vi "Get WS Status.vi"(4 "Secret ID (Default)":string, 6 "Access ID (Default)":string, 7 "WS Name":string, 8 "error in (no error)":errorcluster, 9 "Port":u16, 10 "Host":string, 11 "Scheme (HTTP)":T2) -> (0 "error out":errorcluster, 3 "Status":T1)   [LabVIEW 2020, in "WS Admin.lvlib"]
uses:
  WS Admin.lvlib
  Scheme.ctl
  WS Status.ctl
  Client Data.ctl
  HTTP Method.ctl
  <vilib>/regexp/Match Regular Expression.xnode
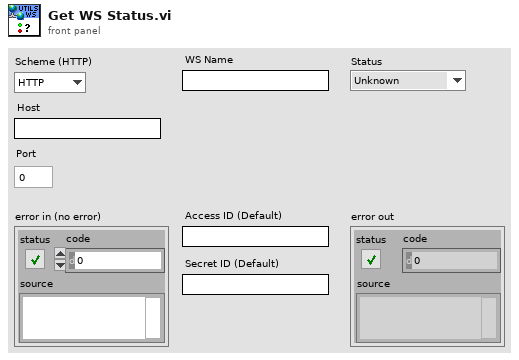
[diagram p1: front panel]
types:
  T1 = typedef "WS Admin.lvlib/WS Status.ctl" = enum16{"Unknown", "Paused", "Running"}
  T2 = typedef "WS Admin.lvlib/Scheme.ctl" = enum16{"HTTP", "HTTPS"}
  T3 = typedef "WS Admin.lvlib/HTTP Method.ctl" = enum16{"GET", "POST", "PUT", "DELETE"}
  T4 = typedef "WS Admin.lvlib/Client Data.ctl" = cluster{"HTTP Method":T3, "URL Path":string, "Access ID":string, "Secret ID":string}
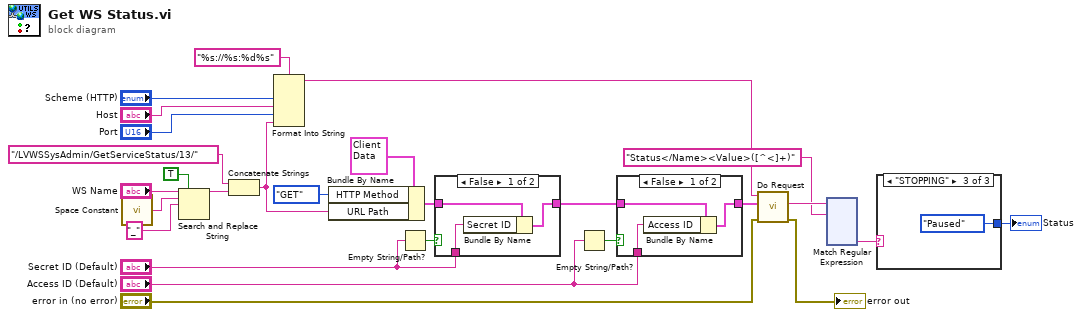
[diagram p0: block diagram]
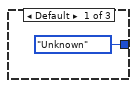
[diagram p2: hidden frame]
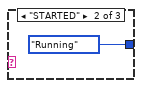
[diagram p3: hidden frame]
diagram:
  n1 = call <vilib>:"Space Constant.vi"() -> ("String"=w26:string)
  n2 = Search and Replace String(replace all?=TRUE ("replace all? (F)"), input string="WS Name", search string=w26, replace string="_" ("replace string (\"\")")) -> (result string=w19:string)  [unwired: 4 in, 3 out]
  n3 = Concatenate Strings("/LVWSSysAdmin/GetServiceStatus/13/", w19) -> (w16:string)
  n4 = Format Into String(format string="%s://%s:%d%s", "Scheme (HTTP)", "Host", "Port", w16) -> (resulting string=w6:string)  [unwired: 2 in, 1 out]
  n5 = Bundle By Name(cluster=T4 {"HTTP Method"=enum."GET", "URL Path"="", "Access ID"="PqVr/ifkAQh+lVrdPIykXlFvg12GhhQFR8H9cUhphgg=", "Secret ID"="pTe9HRlQuMfJxAG6QCGq7UvoUpJzAzWGKy5SbZ+roSU="} ("Client Data"), "HTTP Method"=HTTP_Method."GET", "URL Path"=w16) -> (w13:T4)
  n6 = Empty String/Path?(string/path="Secret ID (Default)") -> (empty?=w14:bool)
  n7 = case shown="False" w14 {
    tunnel: w13 -> [w30 w31]
    tunnel: "Secret ID (Default)" -> [w29 _]
    tunnel: [w28 w31] -> w11
    frame False {
      n8 = Bundle By Name(cluster=w30, "Secret ID"=w29) -> (w28:T4)
    }
    frame True {
    }
  }
  n9 = Empty String/Path?(string/path="Access ID (Default)") -> (empty?=w10:bool)
  n10 = case shown="False" w10 {
    tunnel: w11 -> [w34 w35]
    tunnel: "Access ID (Default)" -> [w33 _]
    tunnel: [w32 w35] -> w8
    frame False {
      n11 = Bundle By Name(cluster=w34, "Access ID"=w33) -> (w32:T4)
    }
    frame True {
    }
  }
  n12 = call "Do Request.vi"("error in (no error)"="error in (no error)", "Client Data"=w8, "URL"=w6) -> ("error out"=→"error out":errorcluster, "Response Body"=w4:string)  [unwired: 7 in]
  n13 = xnode "Match Regular Expression"("input string"=w4, "regular expression"="Status</Name><Value>([^<]+)") -> ("submatch 1"=w2:string)  [unwired: 4 in, 5 out]
  n14 = case shown="\"STOPPING\"" w2 {
    tunnel: [WS_Status."Unknown" ("WS Status") WS_Status."Running" ("WS Status") WS_Status."Paused" ("WS Status")] -> w1
    frame Default {
    }
    frame "STARTED" {
    }
    frame "STOPPING" {
    }
  }
  "Status" <- w1
